vi "Pnuematics Controller.vi"(8 "error in":errorcluster) -> ()   [LabVIEW 2019]
doc: "This VI executes continuously carrying out the current operation and responding to updates or new operations. It will often contain the timing or control code that is difficult to place directly in TeleOp. This VI generally opens all sensors and motors and isolates the rest of the robot code from knowing how the operations are carried out."
uses:
  <vilib>/Rock Robotics/WPI/Framework/Completion Status.ctl
  Pnuematics Setpoints.ctl
  Pnuematics Operations.ctl
  <vilib>/Rock Robotics/WPI/Solenoid/WPI_SolenoidValue.ctl
  <vilib>/Rock Robotics/WPI/Solenoid/WPI_SolenoidChannel.ctl
  <vilib>/Rock Robotics/WPI/Solenoid/WPI_SolenoidOpenDouble.vi
  <vilib>/Rock Robotics/WPI/Solenoid/WPI_SolenoidSetEnum.vi
  <vilib>/Rock Robotics/WPI/Utilities/WPI_GetSetVariantRefNum.vi
  <vilib>/Rock Robotics/Network Tables/NT Write Boolean.vi
panel:
  in  "Interactive Values":T1={"Operation"=enum."Reserve", "Value"=enum."On", "Solenoid"=enum."Transmission", "Milliseconds"=0.0}
  out "Current\nCmd":string
  in  "Buttons":cluster{"Execute Cmd":bool, "Abort Cmd":bool}
  out "Command Timing":cluster{"Start Time (ms)":u32, "Iterations":i32}
  out "Status":T4
  # "Tip: It may be helpful to observe inputs and sensor values.\nYou may also want to display tuning or debugging controls."
  # "Interactive Command: You may fill in the settings for a command\nand schedule it with the Execute button. You can observe and abort\nany command while fine tuning the code for the controller."
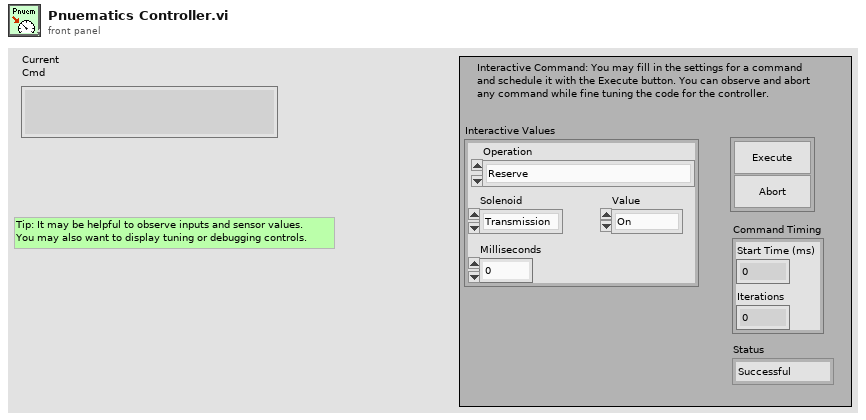
[diagram p1: front panel]
types:
  T1 = typedef "Pnuematics Setpoints.ctl" = cluster{"Operation":T2, "Value":T3, "Solenoid":enum16{"Default", "Transmission", "Wheel"}, "Milliseconds":dbl}
  T2 = typedef "Pnuematics Operations.ctl" = enum16{"Reserve", "Read Current", "CompressorStart", "CompressorEnabled", "CompressorStop", "Solenoid", "Immediate"}
  T3 = typedef "WPI_SolenoidValue.ctl" = enum16{"Off", "On", "Forward", "Reverse"}
  T4 = typedef "Completion Status.ctl" = enum16{"Successful", "Aborted", "Incomplete"}
  T5 = typedef "WPI_SolenoidChannel.ctl" = enum8{"Solenoid 0", "Solenoid 1", "Solenoid 2", "Solenoid 3", "Solenoid 4", "Solenoid 5", "Solenoid 6", "Solenoid 7", "Invalid"}
  T6 = typedef "WPI_SolenoidDevRef.ctl" = cluster{"DevStatus":errorcluster, "Pneumatics Control Module":u8, "Forward Solenoid Channel":T5, "Reverse Solenoid Channel":T5}
  T7 = typedef "WPI_CompressorDevRef.ctl" = cluster{"DevStatus":errorcluster, "Pneumatics Control Module":u8}
  T8 = typedef "Command Status Info.ctl" = cluster{"Name":string, "Status":T4, "notifier out":T9}
  T9 = typedef "Completion Notifier.ctl" = refnum<notifier>
  T10 = cluster{"Current Command":T1, "Command Timing":cluster{"Start Time (ms)":u32, "Iterations":i32}, "Command Arguments":cluster{"Command Info":T8, "Description":string, "Default Command":T1, "queue out":refnum<queue>, "Subsystem Name":string}}
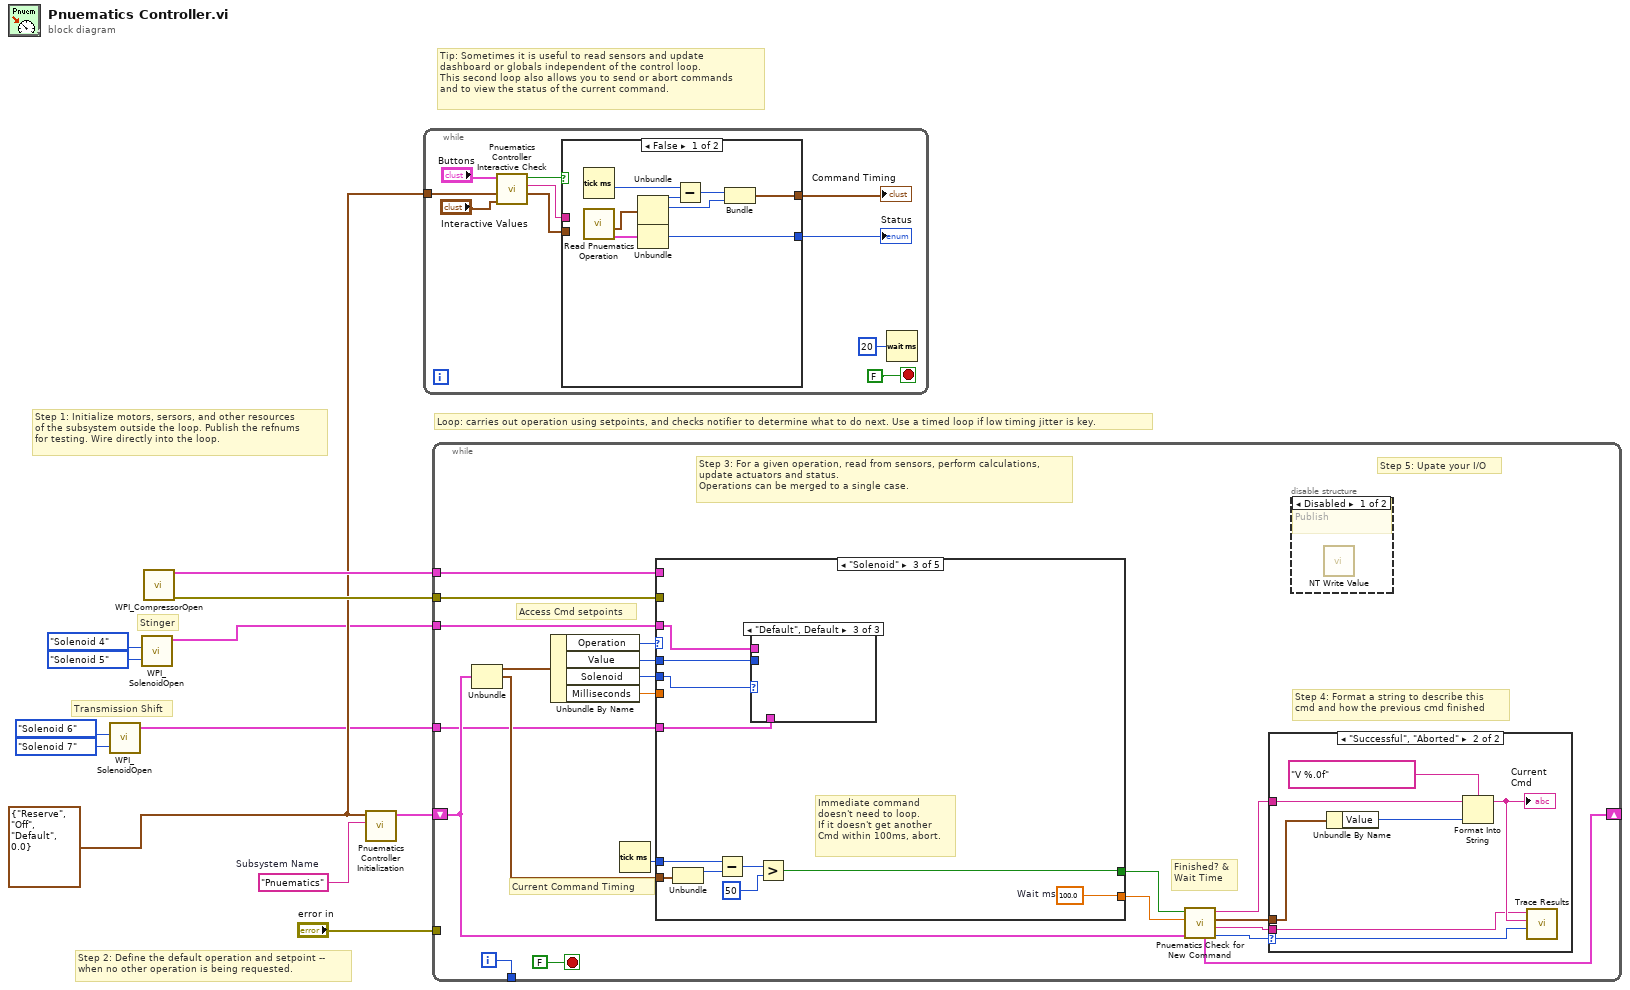
[diagram p0: block diagram]
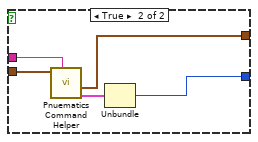
[diagram p2: hidden frame]
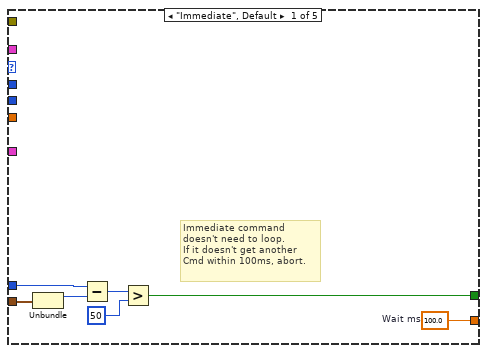
[diagram p5: hidden frame]
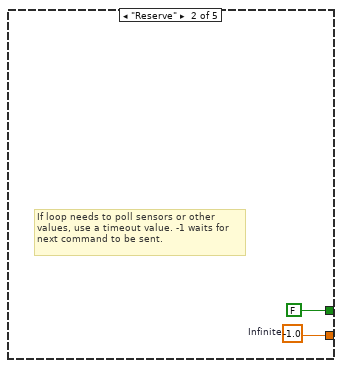
[diagram p6: hidden frame]
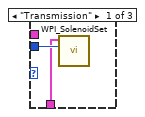
[diagram p7: hidden frame]
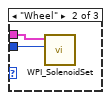
[diagram p8: hidden frame]
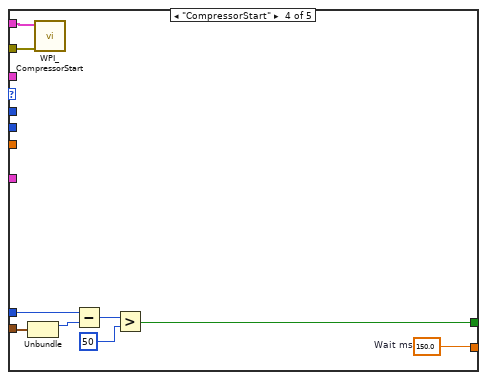
[diagram p9: hidden frame]
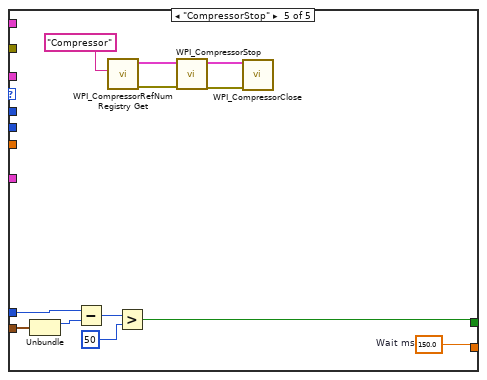
[diagram p10: hidden frame]
diagram:
  w7 = T1 {"Operation"=enum."Reserve", "Value"=enum."Off", "Solenoid"=enum."Default", "Milliseconds"=0.0} ("Default Command")
  w10 = "Pnuematics"  # Subsystem Name
  # "Transmission Shift"
  # "Stinger"
  # "Tip: Sometimes it is useful to read sensors and update\ndashboard or globals independent of the control loop.\nThis second loop also allows you to send or abort commands\nand to view the status of the current command."
  # "Step 2: Define the default operation and setpoint --\nwhen no other operation is being requested."
  # "Step 1: Initialize motors, sersors, and other resources\nof the subsystem outside the loop. Publish the refnums\nfor testing. Wire directly into the loop."
  # "Loop: carries out operation using setpoints, and checks notifier to determine what to do next. Use a timed loop if low timing jitter is key."
  n1 = call-poly <vilib>:"WPI_SolenoidOpen.vi"("Reverse Solenoid Channel"=WPI_SolenoidChannel."Solenoid 7", "Forward Solenoid Channel"=WPI_SolenoidChannel."Solenoid 6") -> ("SolenoidDevRef"=w2:T6)  [unwired: 8 in, 1 out]
  n2 = call-poly <vilib>:"WPI_SolenoidOpen.vi"("Reverse Solenoid Channel"=WPI_SolenoidChannel."Solenoid 5", "Forward Solenoid Channel"=WPI_SolenoidChannel."Solenoid 4") -> ("SolenoidDevRef"=w1:T6)  [unwired: 8 in, 1 out]
  n3 = call <vilib>:"WPI_CompressorOpen.vi"() -> ("CompressorDevRef"=w9:T7, "error out"=w8:errorcluster)  [unwired: 14 in]
  n4 = call "Pnuematics Controller Initialization.vi"("Subsystem Name"=w10, "Default Command"=w7) -> ("Current Command"=w11:T10)  [unwired: 9 in]
  n5 = while {
    tunnel: w7 -> [w19]
    stop <- FALSE stop-if-true
    n6 = call "Pnuematics Controller Interactive Check.vi"("Interactive Command in"="Interactive Values", "Default Command"=w19, "Buttons"="Buttons") -> ("Interactive Command out"=w16:T1, "Trace String"=w17:string, "Schedule"=w18:bool)  [unwired: 6 in]
    n7 = case shown="False" w18 {
      tunnel: [w30 w35] -> w15
      tunnel: w16 -> [_ w33]
      tunnel: [w26 w31] -> w14
      tunnel: w17 -> [_ w34]
      frame False {
        n8 = Tick Count (ms)() -> (millisecond timer value=w25:u32)
        n9 = call "Read Pnuematics Operation.vi"() -> ("Command Info"=w23:T8, "SubSystem Data"=w24:T1)  [unwired: 9 in, 1 out]
        n10 = Unbundle(w24) -> ("Operation"=w29:T2, "Value"=w27:T3)  [unwired: 2 out]
        n11 = Unbundle(w23) -> ("Status"=w30:T4)  [unwired: 2 out]
        n12 = Subtract(x=w25, y=w29) -> (x-y=w28:u32)
        n13 = Bundle(w28, "Value"=w27) -> (w26:cluster{u32, "Value":T3})  [unwired: 1 in]
      }
      frame True {
        n14 = call "Pnuematics Command Helper.vi"("Description"=w34, "SubSystem Data"=w33) -> ("Command Info Out"=w32:T8, "Command Timing"=w31:cluster{"Start Time (ms)":u32, "Iterations":i32})  [unwired: 7 in, 1 out]
        n15 = Unbundle(w32) -> ("Status"=w35:T4)  [unwired: 2 out]
      }
    }
    "Status" <- w15
    "Command Timing" <- w14
    n16 = Wait (ms)(milliseconds to wait=u32 20) -> ()  [unwired: 1 out]
  }
  n17 = while {
    shift-right: [w49] -> _
    shift-left: w11 -> [w42]
    tunnel: [w55] -> _
    tunnel: "error in" -> [_]
    tunnel: w9 -> [w40]
    tunnel: w8 -> [w39]
    tunnel: w1 -> [w37]
    tunnel: w2 -> [w36]
    i -> [w55]
    stop <- FALSE stop-if-true
    # "Step 5: Upate your I/O"
    # "Step 4: Format a string to describe this\ncmd and how the previous cmd finished"
    # "Current Command Timing"
    # "Access Cmd setpoints"
    # "Finished? &\nWait Time"
    # "Step 3: For a given operation, read from sensors, perform calculations,\nupdate actuators and status.\nOperations can be merged to a single case."
    n18 = Unbundle(w42) -> ("Current Command"=w54:T1, "Command Timing"=w50:cluster{"Start Time (ms)":u32, "Iterations":i32})  [unwired: 1 out]
    n19 = Unbundle By Name(w54) -> ("Operation"=w53:T2, "Value"=w52:T3, "Solenoid"=w41:enum16{"Default", "Transmission", "Wheel"}, "Milliseconds"=w38:dbl)
    n20 = Tick Count (ms)() -> (millisecond timer value=w51:u32)
    n21 = case shown="\"Solenoid\"" w53 {
      tunnel: [w70 w72 w77 w91 w100] -> w47
      tunnel: [w64 FALSE ("ignore previous (F)") w78 w90 w101] -> w48
      tunnel: w50 -> [w66 _ w80 w93 w103]
      tunnel: w52 -> [_ _ w76 _ _]
      tunnel: w51 -> [w65 _ w79 w92 w102]
      tunnel: w41 -> [_ _ w75 _ _]
      tunnel: w40 -> [_ _ _ w89 _]
      tunnel: w39 -> [_ _ _ w88 _]
      tunnel: w38 -> [_ _ _ _ _]
      tunnel: w37 -> [_ _ w74 _ _]
      tunnel: w36 -> [_ _ w73 _ _]
      frame "Immediate", Default {
        w70 = 100.0  # Wait ms
        # "Immediate command\ndoesn't need to loop.\nIf it doesn't get another\nCmd within 100ms, abort."
        n22 = Unbundle(w66) -> ("Start Time (ms)"=w69:u32)  [unwired: 1 out]
        n23 = Subtract(x=w65, y=w69) -> (x-y=w68:u32)
        n24 = Greater?(x=w68, y=u8 50 ("Left Motor")) -> (0:w64:bool)
      }
      frame "Reserve" {
        w72 = -1.0  # Infinite
        # "If loop needs to poll sensors or other\nvalues, use a timeout value. -1 waits for\nnext command to be sent."
      }
      frame "Solenoid" {
        w77 = 100.0  # Wait ms
        # "Immediate command\ndoesn't need to loop.\nIf it doesn't get another\nCmd within 100ms, abort."
        n25 = Unbundle(w80) -> ("Start Time (ms)"=w83:u32)  [unwired: 1 out]
        n26 = Subtract(x=w79, y=w83) -> (x-y=w82:u32)
        n27 = case shown="\"Default\", Default" w75 {
          tunnel: w76 -> [w85 w87 _]
          tunnel: w74 -> [_ w86 _]
          tunnel: w73 -> [w84 _ _]
          frame "Transmission" {
            n28 = call-poly <vilib>:"WPI_SolenoidSet.vi"("Value"=w85, "SolenoidDevRef"=w84) -> ()  [unwired: 8 in, 2 out]
          }
          frame "Wheel" {
            n29 = call-poly <vilib>:"WPI_SolenoidSet.vi"("Value"=w87, "SolenoidDevRef"=w86) -> ()  [unwired: 8 in, 2 out]
          }
          frame "Default", Default {
          }
        }
        n30 = Greater?(x=w82, y=u8 50 ("Left Motor")) -> (0:w78:bool)
      }
      frame "CompressorStart" {
        w91 = 150.0  # Wait ms
        n31 = Unbundle(w93) -> ("Start Time (ms)"=w94:u32)  [unwired: 1 out]
        n32 = call <vilib>:"WPI_CompressorStart.vi"("error in (no error)"=w88, "CompressorDevRef"=w89) -> ()  [unwired: 8 in, 2 out]
        n33 = Subtract(x=w92, y=w94) -> (x-y=w96:u32)
        n34 = Greater?(x=w96, y=u8 50 ("Left Motor")) -> (0:w90:bool)
      }
      frame "CompressorStop" {
        w100 = 150.0  # Wait ms
        n35 = Unbundle(w103) -> ("Start Time (ms)"=w104:u32)  [unwired: 1 out]
        n36 = Subtract(x=w102, y=w104) -> (x-y=w106:u32)
        n37 = call <vilib>:"WPI_CompressorRefNum Registry Get.vi"("refnum name"="Compressor") -> ("error out"=w99:errorcluster, "CompressorDevRef"=w108:T7)  [unwired: 9 in]
        n38 = Greater?(x=w106, y=u8 50 ("Left Motor")) -> (0:w101:bool)
        n39 = call <vilib>:"WPI_CompressorStop.vi"("error in (no error)"=w99, "CompressorDevRef"=w108) -> ("error out"=w97:errorcluster, "CompressorDevRef"=w98:T7)  [unwired: 8 in]
        n40 = call <vilib>:"WPI_CompressorClose.vi"("error in (no error)"=w97, "CompressorDevRef"=w98) -> ()  [unwired: 9 in, 1 out]
      }
    }
    n41 = call "Pnuematics Check for New Command.vi"("Current Command"=w42, "Wait time (ms)"=w47, "Finished?"=w48) -> ("Completion"=w43:T4, "Subsystem Name"=w44:string, "Current Command"=w45:T1, "Initial Trace String"=w46:string, "NextCommand"=w49:T10)  [unwired: 4 in]
    n42 = case shown="\"Successful\", \"Aborted\"" w43 {
      selector: w43 -> [_ w63]
      tunnel: w46 -> [_ w59]
      tunnel: w45 -> [_ w60]
      tunnel: w44 -> [_ w57]
      frame "Incomplete", Default {
        # "Continuing current command"
      }
      frame "Successful", "Aborted" {
        # "Report and setup for next command"
        n43 = Unbundle By Name(w60) -> ("Value"=w62:T3)
        n44 = Format Into String(format string="V %.0f", initial string=w59, w62) -> (resulting string=w58:string)  [unwired: 1 in, 1 out]
        "Current\nCmd" <- w58
        n45 = call <vilib>:"Trace Results.vi"("Status of previous command"=w63, "Description"=w58, "Subsystem"=w57) -> ()  [unwired: 9 in]
      }
    }
    n46 = disable-structure shown="Disabled" {
      frame Disabled {
        # "Publish"
        n47 = call-poly <vilib>:"NT Write Value.vi"() -> ()  [unwired: 11 in, 1 out]
      }
      frame Enabled {
      }
    }
  }
